vi "Array2Tree.vi"(8 "颜色符号列表":cluster{"项名":string, "颜色":u32, "符号":i32}[](array[cluster]), 9 "循环数组":string[](array[string]), 11 "循环树形引用输入":refnum<vi>) -> (0 "错误输出":errorcluster, 3 "循环树形引用输出":refnum<vi>)   [LabVIEW 2020, in "Curve Editor.lvlib"]
uses:
  Curve Editor.lvlib
  Key Value/Key Value.lvlib
panel:
  # "将数组转换为树形"
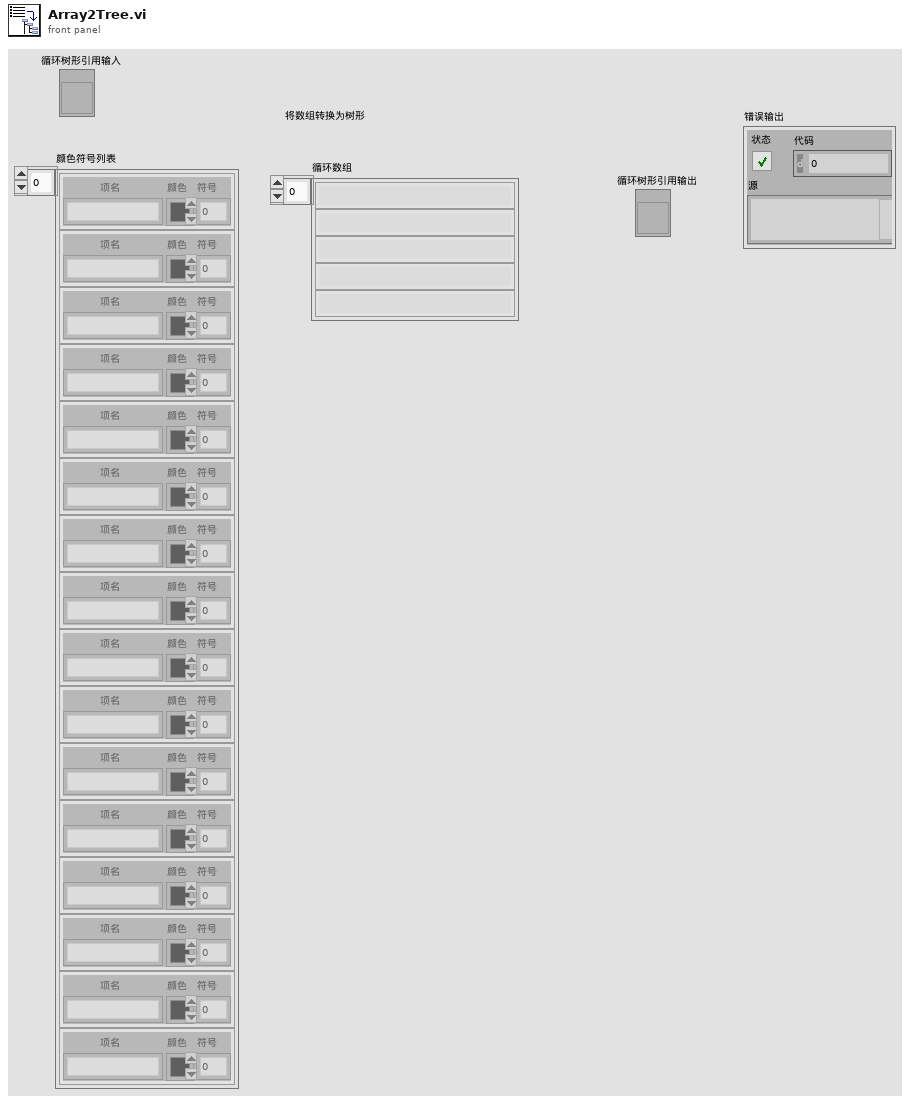
[diagram p1: front panel]
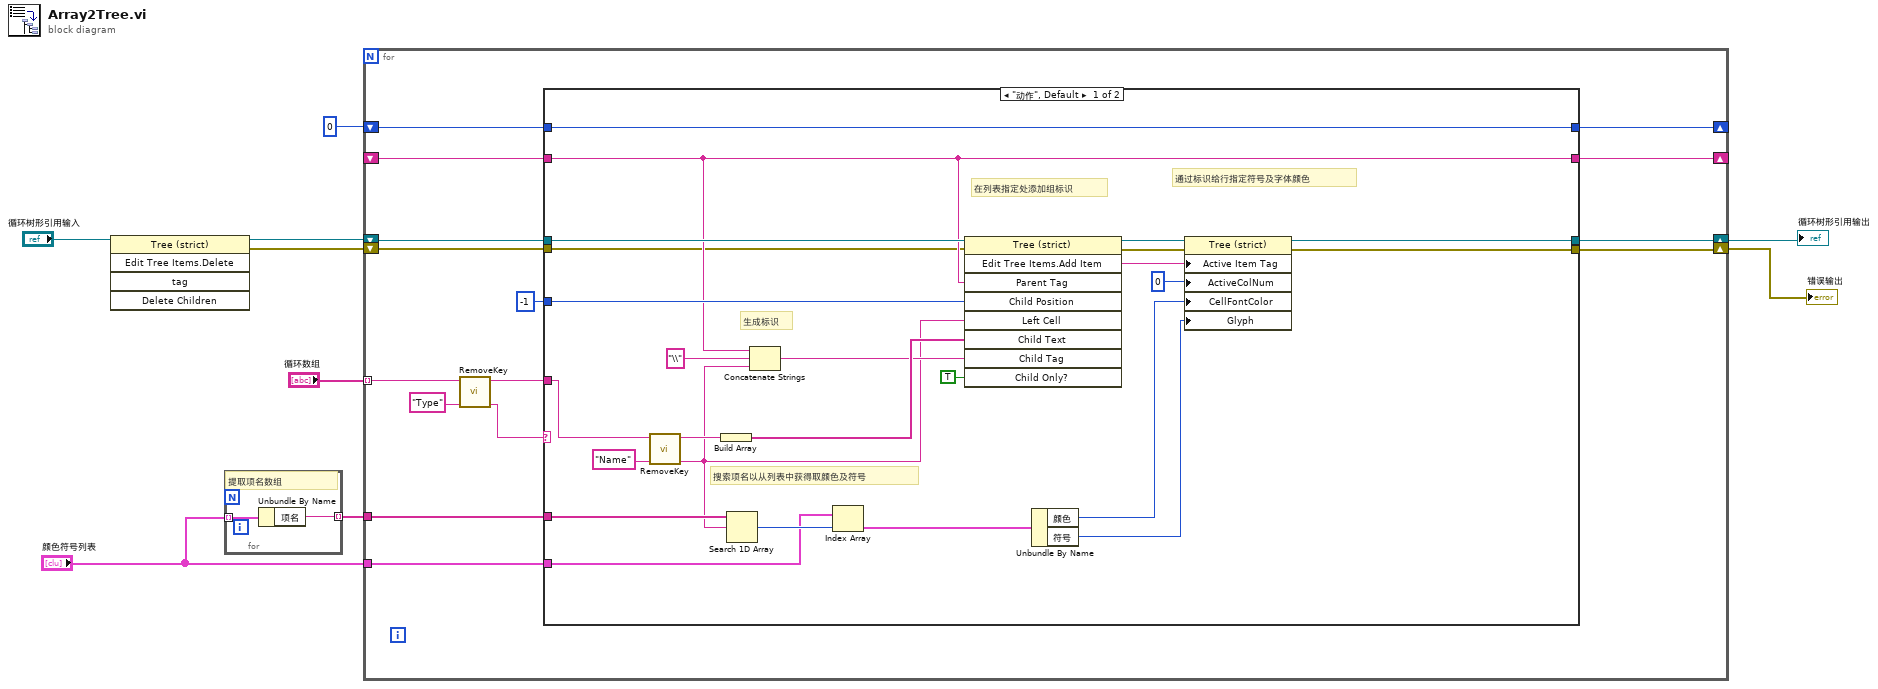
[diagram p0: block diagram]
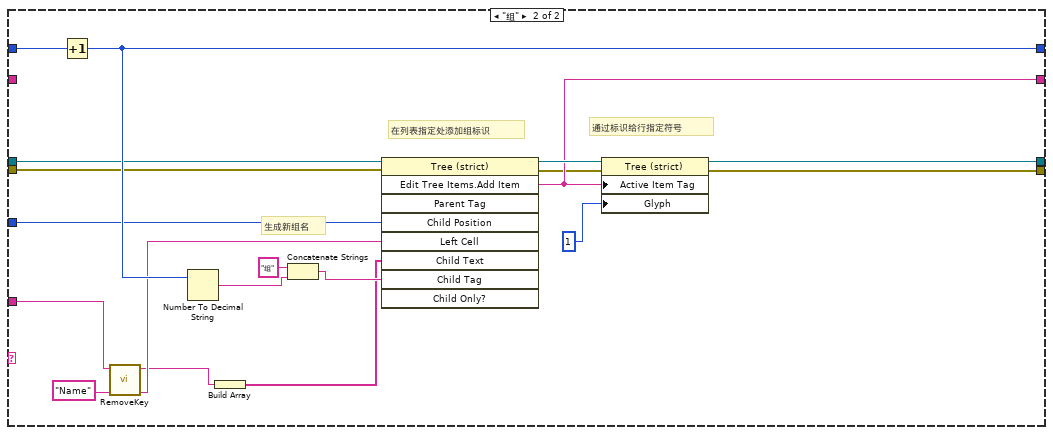
[diagram p2: hidden frame]
diagram:
  n1 = invoke class="Tree (strict)" method="Edit Tree Items.Delete"(reference="循环树形引用输入") -> (reference out=w6:refnum<vi>, error out=w5:errorcluster)  [unwired: 4 in, 3 out]
  n2 = for {
    tunnel: "颜色符号列表" -> [w11] mode=indexing
    tunnel: [w10] -> w7 mode=indexing
    # "提取项名数组"
    n3 = Unbundle By Name(w11) -> ("项名"=w10:string)
  }
  n4 = for {
    tunnel: "循环数组" -> [w19] mode=indexing
    shift-right: [w22] -> _
    shift-left: 0 -> [w23]
    shift-right: [w21] -> _
    shift-left: _ -> [w20]
    tunnel: "颜色符号列表" -> [w17]
    tunnel: w7 -> [w16]
    shift-right: [w15] -> w4
    shift-left: w6 -> [w24]
    shift-right: [w13] -> w3
    shift-left: w5 -> [w14]
    n5 = call "RemoveKey.vi"("键"="Type", "键值串"=w19) -> ("删除的值"=w25:string, "删除后的键值串"=w18:string)  [unwired: 8 in]
    n6 = case shown="\"动作\", Default" w25 {
      tunnel: w24 -> [w48 w62]
      tunnel: w23 -> [w51 w70]
      tunnel: [w51 w65] -> w22
      tunnel: -1 ("x") -> [w47 w63]
      tunnel: [w41 w61] -> w21
      tunnel: w20 -> [w41 _]
      tunnel: w18 -> [w44 w56]
      tunnel: w17 -> [w34 _]
      tunnel: w16 -> [w37 _]
      tunnel: [w30 w55] -> w15
      tunnel: w14 -> [w29 w54]
      tunnel: [w27 w52] -> w13
      frame "动作", Default {
        # "搜索项名以从列表中获得取颜色及符号"
        # "生成标识"
        # "通过标识给行指定符号及字体颜色"
        # "在列表指定处添加组标识"
        n7 = call "RemoveKey.vi"("键"="Name", "键值串"=w44) -> ("删除的值"=w36:string, "删除后的键值串"=w45:string)  [unwired: 8 in]
        n8 = Build Array(w45) -> (w43:string[])
        n9 = Search 1D Array(1D array=w37, element=w36) -> (index of element=w35:i32)  [unwired: 1 in]
        n10 = Concatenate Strings(w41, "\\" ("字符串"), w36) -> (w39:string)
        n11 = Index Array(array=w34, index=w35) -> (element=w33:cluster{"项名":string, "颜色":u32, "符号":i32})
        n12 = invoke class="Tree (strict)" method="Edit Tree Items.Add Item"(reference=w48, error in=w29, "Parent Tag"=w41, "Child Position"=w47, "Left Cell"=w36, "Child Text"=w43, "Child Tag"=w39, "Child Only?"=TRUE ("仅作为子项？")) -> (reference out=w50:refnum<vi>, error out=w28:errorcluster, "Edit Tree Items:Add Item"=w49:string)  [unwired: 1 in, 6 out]
        n13 = Unbundle By Name(w33) -> ("颜色"=w32:u32, "符号"=w31:i32)
        n14 = property class="Tree (strict)"(reference=w50, error in=w28, "Active Item Tag"=w49, "ActiveColNum"=0 ("活动单元格:活动列数"), "CellFontColor"=w32, "Glyph"=w31) -> (reference out=w30:refnum<vi>, error out=w27:errorcluster)
      }
      frame "组" {
        # "通过标识给行指定符号"
        # "在列表指定处添加组标识"
        # "生成新组名"
        n15 = Increment(x=w70) -> (x+1=w65:i32)
        n16 = call "RemoveKey.vi"("键"="Name", "键值串"=w56) -> ("删除的值"=w59:string, "删除后的键值串"=w58:string)  [unwired: 8 in]
        n17 = Number To Decimal String(number=w65) -> (decimal integer string=w64:string)  [unwired: 1 in]
        n18 = Build Array(w58) -> (w57:string[])
        n19 = Concatenate Strings("组" ("字符串"), w64) -> (w67:string)
        n20 = invoke class="Tree (strict)" method="Edit Tree Items.Add Item"(reference=w62, error in=w54, "Child Position"=w63, "Left Cell"=w59, "Child Text"=w57, "Child Tag"=w67) -> (reference out=w68:refnum<vi>, error out=w53:errorcluster, "Edit Tree Items:Add Item"=w61:string)  [unwired: 3 in, 6 out]
        n21 = property class="Tree (strict)"(reference=w68, error in=w53, "Active Item Tag"=w61, "Glyph"=1 ("活动项:符号索引")) -> (reference out=w55:refnum<vi>, error out=w52:errorcluster)
      }
    }
  }
  "循环树形引用输出" <- w4
  "错误输出" <- w3
